vi "ArbitraryFrequency.vi"() -> ()   [LabVIEW 2015]
panel:
  in  "arbitrary frequency":dbl
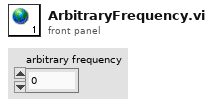
[diagram p1: front panel]
diagram:
